vi "ograniczenie.vi"(6 "dokladnosc":dbl, 11 "Array in":dbl[](array[numeric])) -> (3 "Array":dbl[](array[numeric]))   [LabVIEW 2014]
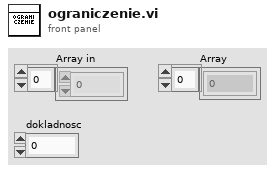
[diagram p1: front panel]
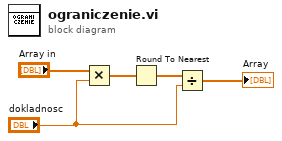
[diagram p0: block diagram]
diagram:
  n1 = Multiply(x="Array in", y="dokladnosc") -> (x*y=w2:dbl[])
  n2 = Round To Nearest(number=w2) -> (nearest integer value=w1:dbl[])
  n3 = Divide(x=w1, y="dokladnosc") -> (x/y=→"Array":dbl[])
